vi "GenerateMeasurementFiles.vi"() -> ()   [LabVIEW 2016]
uses:
  Global/ApplicationGlobal.vi
panel:
  out "Array":errorcluster[](array[cluster])
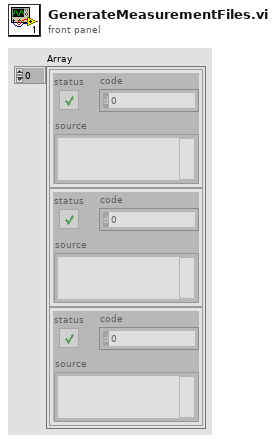
[diagram p1: front panel]
types:
  T1 = enum16{"open", "replace", "create", "open or create", "replace or create", "replace or create with confirmation"}
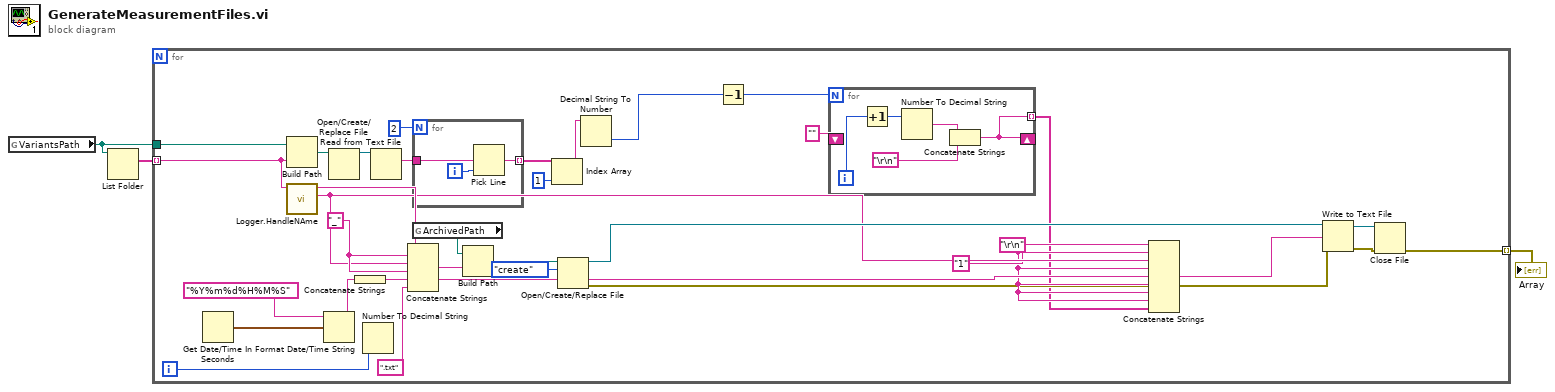
[diagram p0: block diagram]
diagram:
  n1 = global read "ApplicationGlobal.vi" "VariantsPath"() -> (w2:path)
  n2 = List Folder(path=w2) -> (filenames=w3:string[])  [unwired: 3 in, 3 out]
  n3 = for {
    tunnel: w3 -> [w36] mode=indexing
    tunnel: w2 -> [w37]
    tunnel: [w7] -> w1 mode=indexing
    i -> [w22]
    w10 = "\r\n"
    w26 = "_" ("string")
    n4 = Get Date/Time In Seconds() -> (seconds since 1Jan1904=w25:timestamp)
    n5 = Build Path(base path=w37, name or relative path=w36) -> (appended path=w35:path)
    n6 = call "Logger.HandleNAme.vi"("String"=w36) -> ("Variant"=w18:string, "System"=w27:string)  [unwired: 8 in, 1 out]
    n7 = Format Date/Time String(time format string (%c)="%Y%m%d%H%M%S", seconds (now)=w25) -> (date/time string=w17:string)  [unwired: 1 in]
    n8 = Open/Create/Replace File(file path (use dialog)=w35) -> (refnum out=w34:refnum<file>)  [unwired: 5 in, 2 out]
    n9 = Concatenate Strings(w17) -> (w16:string)
    n10 = Number To Decimal String(number=w22) -> ()  [unwired: 1 in, 1 out]
    n11 = Read from Text File(file (use dialog)=w34) -> (text=w33:string)  [unwired: 3 in, 3 out]
    n12 = Concatenate Strings(w27, w26, w18, w26, w16, ".txt" ("string")) -> (w23:string)
    n13 = for {
      N: 2 -> [_]
      tunnel: w33 -> [w43]
      tunnel: [w45] -> w31 mode=indexing
      i -> [w44]
      n14 = Pick Line(multi-line string=w43, line index=w44) -> (output string=w45:string)  [unwired: 1 in]
    }
    n15 = global read "ApplicationGlobal.vi" "ArchivedPath"() -> (w28:path)
    n16 = Build Path(base path=w28, name or relative path=w23) -> (appended path=w20:path)
    n17 = Index Array(array=w31, index=1) -> (element=w29:string)
    n18 = Open/Create/Replace File(file path (use dialog)=w20, operation (0:open)=T1."create") -> (refnum out=w19:refnum<file>, error out=w9:errorcluster)  [unwired: 4 in, 1 out]
    n19 = Decimal String To Number(string=w29) -> (number=w14:i32)  [unwired: 2 in, 1 out]
    n20 = Decrement(x=w14) -> (x-1=w4:i32)
    n21 = for {
      N: w4 -> [_]
      shift-right: [w39] -> _
      shift-left: "" -> [_]
      tunnel: [w39] -> w5 mode=indexing
      i -> [w42]
      n22 = Increment(x=w42) -> (x+1=w38:i32)
      n23 = Number To Decimal String(number=w38) -> (decimal integer string=w41:string)  [unwired: 1 in]
      n24 = Concatenate Strings(w41, "\r\n") -> (w39:string)
    }
    n25 = Concatenate Strings("1", w10, w18, w10, w16, w10, w10, w10, w5) -> (w12:string)
    n26 = Write to Text File(file (use dialog)=w19, text=w12, error in=w9) -> (refnum out=w11:refnum<file>, error out=w8:errorcluster)  [unwired: 1 in, 1 out]
    n27 = Close File(refnum=w11, error in=w8) -> (error out=w7:errorcluster)  [unwired: 1 out]
  }
  "Array" <- w1
